vi "Clone and Open LVLib.vi"(9 "Output LVLib Name":string, 10 "Output LVLib Dir":path, 11 "Template LVLib Path":path) -> (2 "New LVLib":refnum<vi>, 3 "Template LVLib":refnum<vi>)   [LabVIEW 2013]
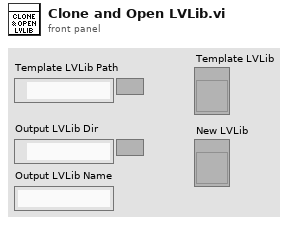
[diagram p1: front panel]
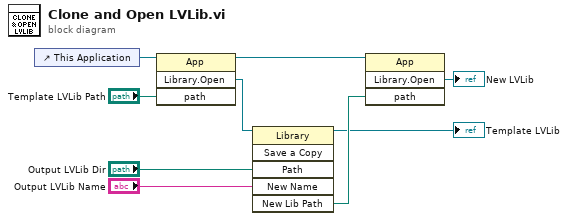
[diagram p0: block diagram]
diagram:
  n1 = control-ref of="This Application"() -> (w5:refnum<vi>)
  n2 = invoke class="App" method="Library.Open"(reference=w5, "path"="Template LVLib Path") -> (reference out=w8:refnum<vi>, "Open Library"=w9:refnum<vi>)  [unwired: 2 in, 2 out]
  n3 = invoke class="Library" method="Save a Copy"(reference=w9, "Path"="Output LVLib Dir", "New Name"="Output LVLib Name") -> (reference out=→"Template LVLib":refnum<vi>, "New Lib Path"=w7:path)  [unwired: 3 in, 4 out]
  n4 = invoke class="App" method="Library.Open"(reference=w8, "path"=w7) -> ("Open Library"=→"New LVLib":refnum<vi>)  [unwired: 2 in, 3 out]
